vi "new Room.vi"(8 "error in (no error)":errorcluster, 10 "roomNumber":i32) -> (0 "error out":errorcluster, 3 "Room* out":refnum<data-value>)   [LabVIEW 2016, in "Room.lvclass"]
uses:
  Room.lvclass
  Room.lvclass/Room.ctl
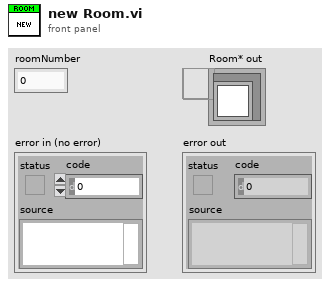
[diagram p1: front panel]
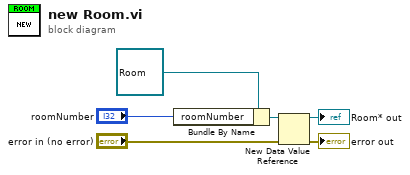
[diagram p0: block diagram]
diagram:
  n1 = Bundle By Name(cluster=refnum<class "Room.lvclass"> refnum ("Room in"), "roomNumber"="roomNumber") -> (w4:refnum<class "Room.lvclass">)
  n2 = New Data Value Reference(data value=w4, error in="error in (no error)") -> (data value reference=→"Room* out":refnum<data-value>, error out=→"error out":errorcluster)
